vi "Nota de VF.vi"(10 "VC":dbl, 11 "VEs":dbl[](array[numeric])) -> (3 "VF":dbl)   [LabVIEW 2018]
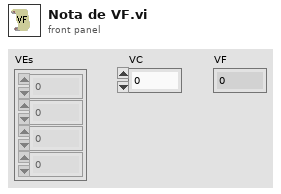
[diagram p1: front panel]
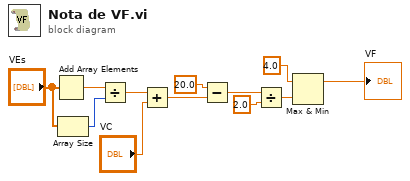
[diagram p0: block diagram]
diagram:
  n1 = Add Array Elements(numeric array="VEs") -> (sum=w1:dbl)
  n2 = Array Size(array="VEs") -> (size(s)=w3:i32)
  n3 = Divide(x=w1, y=w3) -> (x/y=w11:dbl)
  n4 = Add(x=w11, y="VC") -> (x+y=w9:dbl)
  n5 = Subtract(x=20.0, y=w9) -> (x-y=w8:dbl)
  n6 = Divide(x=w8, y=2.0) -> (x/y=w4:dbl)
  n7 = Max & Min(x=4.0, y=w4) -> (max(x,y)=→"VF":dbl)  [unwired: 1 out]
